vi "TEST - Dist Build App from LLB (proxy).vi"(8 "error in (no error)":errorcluster) -> (0 "error out":errorcluster, 2 "pass":bool)   [LabVIEW 2009]
uses:
  <userlib>/_OpenG.lib/file/file.llb/Convert File Extension (Path)__ogtk.vi
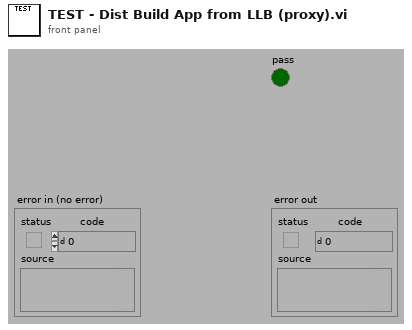
[diagram p1: front panel]
types:
  T1 = cluster{"destination executable":path, "source llb":path, "source shell":path, "custom icon":path}
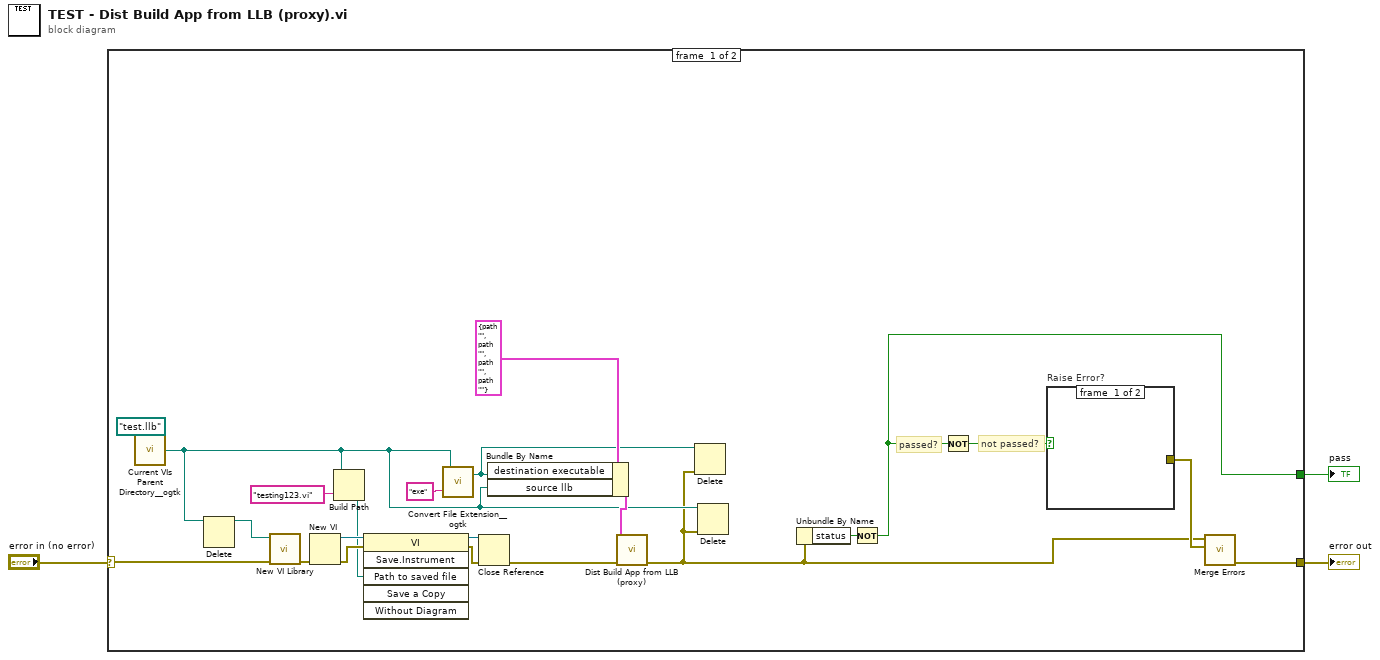
[diagram p0: block diagram]
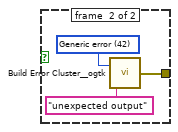
[diagram p2: hidden frame]
diagram:
  n1 = case shown="No Error" "error in (no error)" {
    selector: "error in (no error)" -> [w14 w29]
    tunnel: [w8 _] -> w3
    tunnel: [w25 w29] -> w1
    frame #0 {
      # "not passed?"
      # "passed?"
      n2 = call <userlib>:"Current VIs Parent Directory__ogtk.vi"("Relative path (.)"=path "test.llb") -> ("Parent Directory (+ Relative)"=w5:path)  [unwired: 4 in]
      n3 = Delete(path (use dialog)=w5) -> (deleted path=w7:path)  [unwired: 4 in, 2 out]
      n4 = call <vilib>:"New VI Library.vi"("error in (no error)"=w14, "VI library path in"=w7) -> ("error out"=w21:errorcluster)  [unwired: 8 in, 1 out]
      n5 = New VI(8:w21) -> (0:w20:errorcluster, 3:w19:refnum<vi>)  [unwired: 6 in]
      n6 = Build Path(base path=w5, name or relative path="testing123.vi") -> (appended path=w17:path)
      n7 = invoke class="VI" method="Save.Instrument"(reference=w19, error in=w20, "Path to saved file"=w17) -> (reference out=w16:refnum<vi>, error out=w15:errorcluster)  [unwired: 3 in, 4 out]
      n8 = call-poly <userlib>:"Convert File Extension__ogtk.vi"("new ending (none)"="exe", "file name"=w5) -> ("new filename"=w6:path)  [unwired: 1 out]
      n9 = Close Reference(reference=w16, error in (no error)=w15) -> (error out=w13:errorcluster)
      n10 = Bundle By Name(cluster=T1 {"destination executable"=path "", "source llb"=path "", "source shell"=path "", "custom icon"=path ""} ("paths"), "destination executable"=w6, "source llb"=w5) -> (w10:T1)
      n11 = call "Dist Build App from LLB (proxy).vi"("error in"=w13, "paths"=w10) -> ("error out"=w4:errorcluster)  [unwired: 9 in]
      n12 = Delete(path (use dialog)=w6, error in=w4) -> ()  [unwired: 3 in, 3 out]
      n13 = Delete(path (use dialog)=w5, error in=w4) -> ()  [unwired: 3 in, 3 out]
      n14 = Unbundle By Name(w4) -> ("status"=w9:bool)
      n15 = Not(x=w9) -> (.not. x?=w8:bool)
      n16 = Not(x=w8) -> (.not. x?=w23:bool)
      n17 = case "Raise Error?" shown="True" w23 {
        tunnel: [_ w26] -> w24
        frame #0 {
        }
        frame #1 {
          w27 = 42 items=["No error", "Argument error", "Memory is full", "Out of zone", "End of file", "File already open", "Generic file I/O error", "File not found", "File permission error", "Disk is full", "Duplicate path", "Too many files open", "System feature not enabled", "Resource file not found", "Cannot add resource", "Resource not found", "Image not found", "Image memory error", "Pen does not exist", "Config type invalid", "Config token not found", "Config parse error", "Config memory error", "Bad external code format", "Bad external code offset", "External code not present", "Null window", "Destroy window error", "Null menu", "Print aborted", "Bad print record", "Print driver error", "Windows error during printing", "Memory error during printing", "Print dialog error", "Generic print error", "Invalid device refnum", "Device not found", "Device parameter error", "Device unit error", "Cannot open device", "Device call aborted", "Generic error", "Cancelled by user", "Object ID too low", "Object ID too high", "Object not in heap", "Unknown heap", "Unknown object (invalid DefProc)", "Unknown object (DefProc not in table)", "Message out of range", "Invalid (null) method", "Unknown message", "Manager call not supported", "Bad address", "Network operation in progress", "Network operation timed out", "Connection is busy", "Network attribute not supported", "Network error", "Address in use", "System out of memory", "Connection aborted", "Connection refused", "Not connected", "Already connected", "Connection closed", "Initialization error (interapplication manager)", "Bad occurrence", "Wait on unbound occurrence handler", "Occurrence queue overflow", "Datalog type conflict", "Unused", "Unrecognized type (interapplication manager)", "Memory corrupt", "Failed to make temporary DLL", "Old CIN version", "Drag socket not found", "Failed to load drop-object", "Failed to register OLE object", "Failed to release OLE object", "Format specifier type mismatch", "Unknown format specifier", "Too few format specifiers", "Too many format specifiers", "Scan failed", "Newer CIN version", "Error converting to variant", "Runtime menu error", "Password tampered", "Variant attribute not found", "Incompatible variant data type", "Event data is not available", "Event Store is not present", "Occurrence is not found", "Event Queue is not created", "Event info is not available", "Refnum passed is NULL", "Error retrieving Class GUID", "Error retrieving CoClass GUID", "Error retrieving TypeLib GUID.", "Bad built application magic bytes.", "Specific driver is different from the specific driver associated with the Logical Name.", "There is no session opened to the class driver.", "Max Error", "MAX - Error with config objects", "MAX - Error loading configuration", "MAX - Group not supported"]
          n18 = call <userlib>:"Build Error Cluster__ogtk.vi"("String to Prepend to source (\"\")"="unexpected output" ("String to Prepend to source (\"\")"), "code"=w27) -> ("error out"=w26:errorcluster)
        }
      }
      n19 = call <vilib>:"Merge Errors.vi"("error in 2 (no error)"=w24, "error in 1 (no error)"=w4) -> ("error out"=w25:errorcluster)  [unwired: 5 in]
    }
    frame #1 {
    }
  }
  "pass" <- w3
  "error out" <- w1
